vi "Queues vs Local Variables.vi"() -> ()   [LabVIEW 2012]
panel:
  out "Missing Samples":i32
  out "Loop Rate (ms)":u32
  out "Loop Rate (ms)":u32
  out "Duplicated Samples":i32
  out "Samples":i32
  in  "Loop Speed":u32(ring)=50 items=["Same as Producer Loop"=50, "Maximum Speed"=0, "2x as Producer"=25, "1/2 as Producer"=100, "1/20 as Producer"=1000]
  in  "Loop Speed":u32(ring)=50 items=["Same as Producer Loop"=50, "Maximum Speed"=0, "2x as Producer"=25, "1/2 as Producer"=100, "1/20 as Producer"=1000]
  out "Samples in Queue":i32(slide) scale=0.0..1000.0
  in  "stop":bool
  out "Local Variable Loop":dbl(graph) caption="Local Variables Consumer Chart"
  out "Queue Loop":dbl(graph)=-9.510565162951542 caption="Queues Consumer Chart"
  out "Producer Loop":dbl(graph) caption="Producer Loop Chart"
  # "Producer Loop"
  # "Loop Time = 50 ms"
  # "Local Variable Consumer Loop"
  # "Queue Consumer Loop"
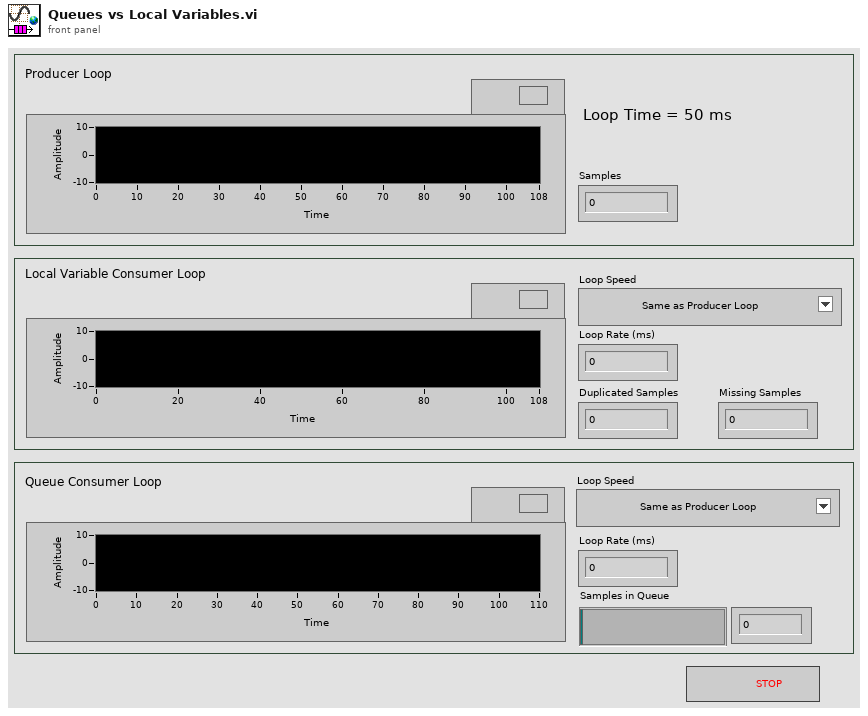
[diagram p1: front panel]
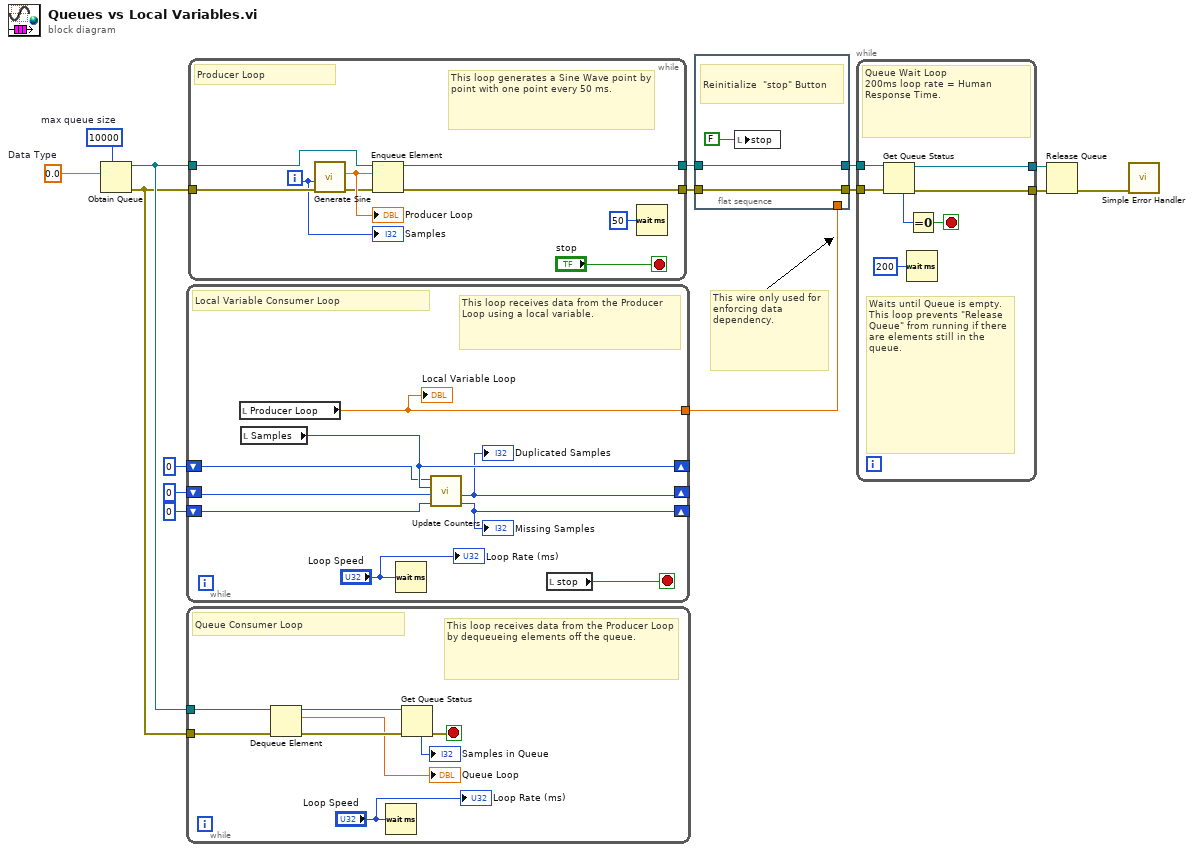
[diagram p0: block diagram]
diagram:
  w1 = 10000  # max queue size
  w15 = 0.0  # Data Type
  # "This wire only used for enforcing data dependency."
  n1 = Obtain Queue(max queue size (-1, unlimited)=w1, element data type=w15) -> (queue out=w14:refnum<queue>, error out=w13:errorcluster)  [unwired: 3 in, 1 out]
  n2 = while {
    tunnel: [w23] -> w5
    shift-right: [w21] -> _
    shift-left: 0 ("Previous Samples") -> [w20]
    shift-right: [w16] -> _
    shift-left: 0 ("Duplicated") -> [w18]
    shift-right: [w19] -> _
    shift-left: 0 ("Missing") -> [w17]
    stop <- w24 stop-if-true
    # "This loop receives data from the Producer Loop using a local variable."
    # "Local Variable Consumer Loop"
    n3 = local read "Producer Loop"() -> (w23:dbl)
    "Local Variable Loop" <- w23
    n4 = local read "Samples"() -> (w21:i32)
    n5 = Wait (ms)(milliseconds to wait="Loop Speed") -> ()  [unwired: 1 out]
    n6 = call "Update Counters.vi"("Current Missing Points"=w17, "Current Duplicated Points"=w18, "Producer Iterations"=w21, "Previous Producer Iterations"=w20) -> ("Updated Missing Points"=w19:i32, "Updated Duplicated Points"=w16:i32)  [unwired: 5 in]
    "Duplicated Samples" <- w16
    "Missing Samples" <- w19
    n7 = local read "stop"() -> (w24:bool)
    "Loop Rate (ms)" <- "Loop Speed"
  }
  n8 = while {
    tunnel: w14 -> [w30]
    tunnel: w13 -> [w29]
    stop <- w27 stop-if-true
    # "This loop receives data from the Producer Loop by dequeueing elements off the queue."
    # "Queue Consumer Loop"
    n9 = Dequeue Element(queue=w30, error in (no error)=w29) -> (queue out=w32:refnum<queue>, element=→"Queue Loop":dbl, error out=w31:errorcluster)  [unwired: 2 out]
    n10 = Wait (ms)(milliseconds to wait="Loop Speed") -> ()  [unwired: 1 out]
    n11 = Get Queue Status(queue=w32, error in (no error)=w31) -> (error out=w27:errorcluster, # elements in queue=→"Samples in Queue":i32)  [unwired: 1 in, 6 out]
    "Loop Rate (ms)" <- "Loop Speed"
  }
  n12 = while {
    tunnel: w14 -> [w35]
    tunnel: w13 -> [w37]
    tunnel: [w40] -> w8
    tunnel: [w39] -> w7
    i -> [w33]
    stop <- "stop" stop-if-true
    # "This loop generates a Sine Wave point by point with one point every 50 ms."
    # "Producer Loop"
    n13 = call "Generate Sine.vi"("Error In"=w37, "Numeric"=w33) -> ("Error Out"=w36:errorcluster, "Sine"=w38:dbl)  [unwired: 1 in, 3 out]
    "Producer Loop" <- w38
    n14 = Enqueue Element(queue=w35, element=w38, error in (no error)=w36) -> (queue out=w39:refnum<queue>, error out=w40:errorcluster)  [unwired: 2 out]
    n15 = Wait (ms)(milliseconds to wait=u32 50) -> ()  [unwired: 1 out]
    "Samples" <- w33
  }
  n16 = flat-sequence {
    tunnel: [w44] -> w9
    tunnel: w8 -> [w44]
    tunnel: w7 -> [w43]
    tunnel: [w43] -> w6
    tunnel: w5 -> [_]
    frame #0 {
      # "Reinitialize  \"stop\" Button"
      n17 = local write "stop"(FALSE ("stop")) -> ()
    }
  }
  n18 = while {
    tunnel: w6 -> [w51]
    tunnel: w9 -> [w50]
    tunnel: [w49] -> w12
    tunnel: [w48] -> w11
    stop <- w46 stop-if-true
    # "Waits until Queue is empty.  This loop prevents \"Release Queue\" from running if there are elements still in the queue."
    # "Queue Wait Loop\n200ms loop rate = Human Response Time."
    n19 = Get Queue Status(queue=w51, error in (no error)=w50) -> (queue out=w48:refnum<queue>, error out=w49:errorcluster, # elements in queue=w47:i32)  [unwired: 6 out]
    n20 = Wait (ms)(milliseconds to wait=u32 200) -> ()  [unwired: 1 out]
    n21 = Equal To 0?(x=w47) -> (x = 0?=w46:bool)
  }
  n22 = Release Queue(queue=w11, error in (no error)=w12) -> (error out=w10:errorcluster)  [unwired: 3 out]
  n23 = call <vilib>:"Simple Error Handler.vi"("error in (no error)"=w10) -> ()  [unwired: 2 in, 7 out]
